vi "setFirstTimestamp.vi"(8 "error in (no error)":errorcluster, 11 "WaveformGenerator in":refnum<class "WaveformGenerator.lvclass">) -> (0 "error out":errorcluster, 3 "WaveformGenerator out":refnum<class "WaveformGenerator.lvclass">)   [LabVIEW 2015, in "WaveformGenerator.lvclass"]
uses:
  WaveformGenerator.lvclass
  WaveformGenerator.lvclass/WaveformGenerator.ctl
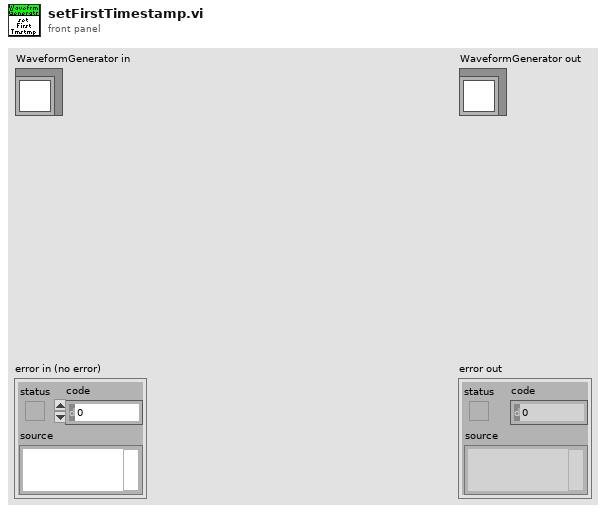
[diagram p1: front panel]
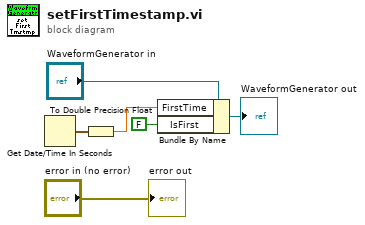
[diagram p0: block diagram]
diagram:
  n1 = Get Date/Time In Seconds() -> (seconds since 1Jan1904=w3:timestamp)
  n2 = To Double Precision Float(number=w3) -> (double precision float=w2:dbl)
  n3 = Bundle By Name(cluster="WaveformGenerator in", "FirstTime"=w2, "IsFirst"=FALSE) -> (→"WaveformGenerator out":refnum<class "WaveformGenerator.lvclass">)
  "error out" <- "error in (no error)"
